vi "LithographyPointsCalculateTime.vi"(8 "error in (no error)":errorcluster, 11 "Asylum_Driver in":refnum<class "Asylum_Driver.lvclass">) -> (0 "error out":errorcluster, 1 "Time":u32, 2 "Interpolation":i32, 3 "Asylum_Driver out":refnum<class "Asylum_Driver.lvclass">)   [LabVIEW 2019, in "Asylum_Driver.lvclass"]
uses:
  Asylum_Driver.lvclass
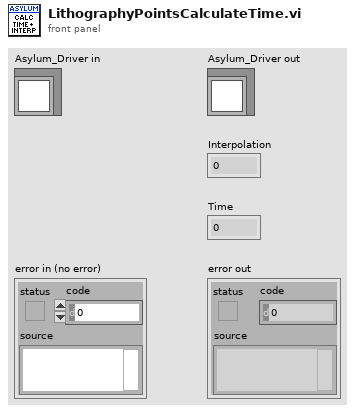
[diagram p1: front panel]
types:
  T1 = typedef "Relay-Box.lvclass/Resistor--enum.ctl" = enum16{"open", "discharge tip", "0 ohms", "100k ohm", "10M ohm", "1G ohm"}
  T2 = cluster{"Name":string, "Litho":cluster{"X":dbl, "Y":dbl, "Speed":dbl, "Voltage":dbl}[], "Set Resistance":T1, "Meta":variant}
  T3 = cluster{"X":dbl, "Y":dbl, "Speed":dbl, "Voltage":dbl}[]
  T4 = cluster{"X":dbl, "Y":dbl, "Speed":dbl, "Voltage":dbl}
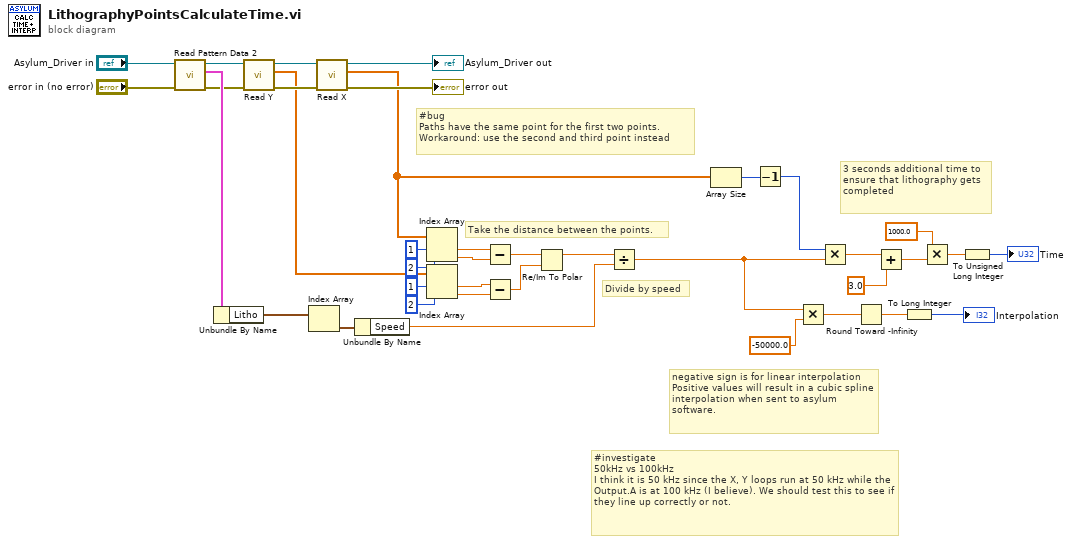
[diagram p0: block diagram]
diagram:
  # "#bug\nPaths have the same point for the first two points. \nWorkaround: use the second and third point instead"
  # "3 seconds additional time to ensure that lithography gets completed"
  # "Divide by speed"
  # "#investigate \n50kHz vs 100kHz\nI think it is 50 kHz since the X, Y loops run at 50 kHz while the Output.A is at 100 kHz (I believe). We should test this to see if they line up correctly or not."
  # "negative sign is for linear interpolation\nPositive values will result in a cubic spline interpolation when sent to asylum software."
  # "Take the distance between the points."
  n1 = call-dynamic "Read Pattern Data 2.vi"("error in (no error)"="error in (no error)", "AFM_Driver in"="Asylum_Driver in") -> ("error out"=w9:errorcluster, "Pattern Data"=w14:T2, "AFM_Driver out"=w10:refnum<class "Asylum_Driver.lvclass">)  [unwired: 7 in]
  n2 = Unbundle By Name(w14) -> ("Litho"=w13:T3)
  n3 = call-dynamic "Read Y.vi"("error in (no error)"=w9, "Asylum_Driver in"=w10) -> ("error out"=w7:errorcluster, "Y"=w4:dbl[], "Asylum_Driver out"=w8:refnum<class "Asylum_Driver.lvclass">)  [unwired: 7 in]
  n4 = Index Array(array=w13) -> (element=w12:T4)  [unwired: 1 in]
  n5 = call-dynamic "Read X.vi"("error in (no error)"=w7, "Asylum_Driver in"=w8) -> ("error out"=→"error out":errorcluster, "X"=w3:dbl[], "Asylum_Driver out"=→"Asylum_Driver out":refnum<class "Asylum_Driver.lvclass">)  [unwired: 7 in]
  n6 = Unbundle By Name(w12) -> ("Speed"=w11:dbl)
  n7 = Index Array(array=w3, index #1=1 ("index"), index #2=2 ("index")) -> (element #1=w38:dbl, element #2=w37:dbl)
  n8 = Index Array(array=w4, index #1=1 ("index"), index #2=2 ("index")) -> (element #1=w36:dbl, element #2=w35:dbl)
  n9 = Subtract(x=w38, y=w37) -> (x-y=w34:dbl)
  n10 = Subtract(x=w36, y=w35) -> (x-y=w33:dbl)
  n11 = Re/Im To Polar(2:w33, 3:w34) -> (1:w32:dbl)  [unwired: 1 out]
  n12 = Divide(x=w32, y=w11) -> (x/y=w30:dbl)
  n13 = Array Size(array=w3) -> (size(s)=w25:i32)
  n14 = Decrement(x=w25) -> (x-1=w24:i32)
  n15 = Multiply(x=w30, y=-50000.0) -> (x*y=w21:dbl)
  n16 = Multiply(x=w24, y=w30) -> (x*y=w23:dbl)
  n17 = Round Toward -Infinity(1:w21) -> (0:w20:dbl)
  n18 = Add(x=w23, y=3.0) -> (x+y=w18:dbl)
  n19 = To Long Integer(number=w20) -> (32bit integer=→"Interpolation":i32)
  n20 = Multiply(x=1000.0, y=w18) -> (x*y=w2:dbl)
  n21 = To Unsigned Long Integer(number=w2) -> (unsigned 32bit integer=→"Time":u32)
